vi "write_buffer_to_file.vi"(8 "error in (no error)":errorcluster, 10 "data_logger.lvclass":refnum<class "data_logger.lvclass">, 11 "tt20 in":refnum<class "tt20.lvclass">) -> (0 "error out":errorcluster, 1 "Stream_done":bool, 2 "data_logger.lvclass_out":refnum<class "data_logger.lvclass">, 3 "tt20 out":refnum<class "tt20.lvclass">)   [LabVIEW 2015, in "tt20.lvclass"]
uses:
  tt20.lvclass
  Data Logger Class/data_logger.lvclass
  tt20.lvclass/tt20.ctl
  C:/Users/MX-Microscope/Documents/LabVIEW Data/lvoop_campus_2018/Detector_Class/Swabian/time_tagger_vis/TTCSharp32.dll
  time_tagger_vis/TTCSharp32.dll
  lvoop_dll-master/picoquant_Tmodes.ctl
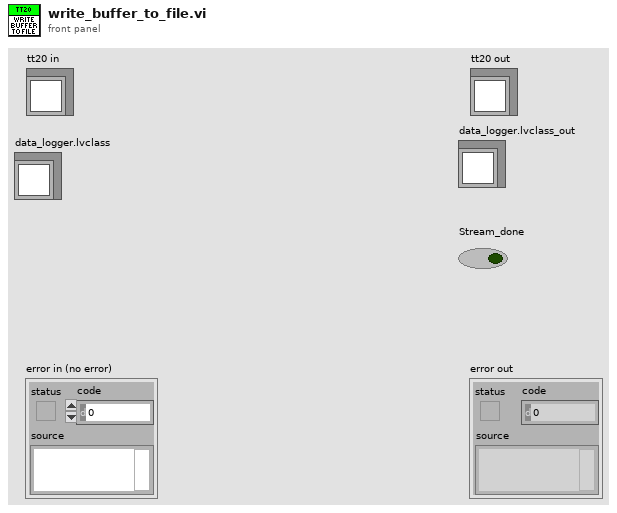
[diagram p1: front panel]
types:
  T1 = typedef "tt20_buffer_tdef.ctl" = cluster{"tagChannels":u32[], "tagTimestamps":i64[], "size":i32}
  T2 = typedef "picoquant_Tmodes.ctl" = u16
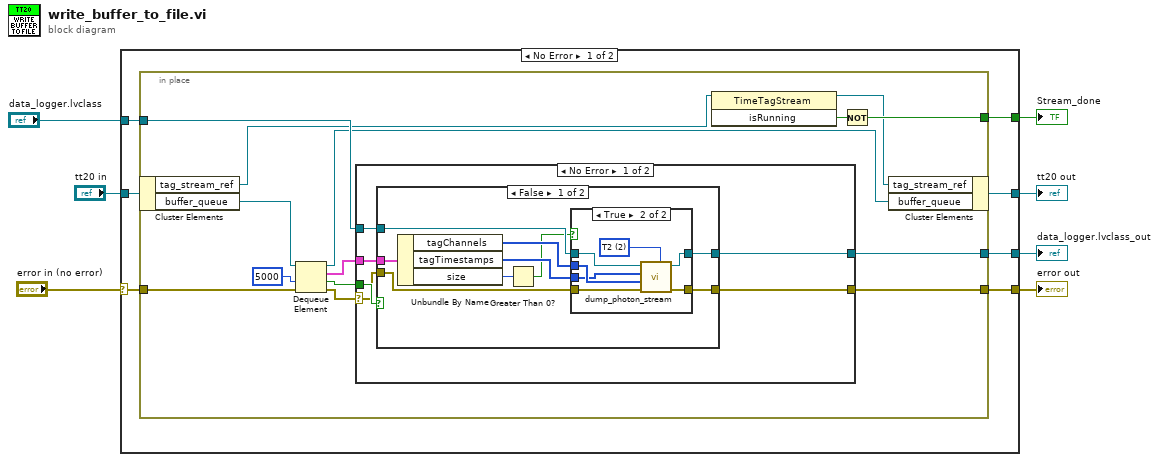
[diagram p0: block diagram]
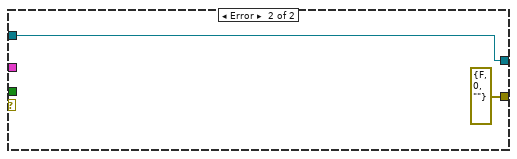
[diagram p4: hidden frame]
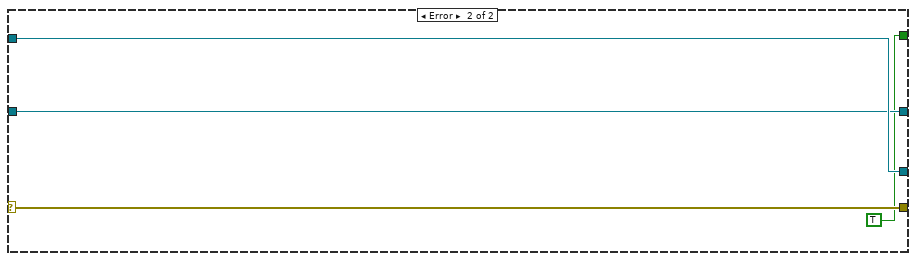
[diagram p5: hidden frame]
diagram:
  n1 = case shown="No Error" "error in (no error)" {
    selector: "error in (no error)" -> [w10 w60]
    tunnel: "tt20 in" -> [w14 w58]
    tunnel: [w13 w58] -> w5
    tunnel: "data_logger.lvclass" -> [w12 w59]
    tunnel: [w11 w59] -> w3
    tunnel: [w9 TRUE] -> w2
    tunnel: [w8 w60] -> w1
    frame No Error {
      n2 = in-place {
        in-place-border: w12 -> [w28]
        in-place-border: [w27] -> w11
        in-place-border: w10 -> [w25]
        in-place-border: [w18] -> w9
        in-place-border: [w17] -> w8
        n3 = in-place-cluster #1(w14) -> ("tag_stream_ref"=w20:refnum<k24>, "buffer_queue"=w26:refnum<queue>)
        n4 = Dequeue Element(queue=w26, timeout in ms (-1)=5000, error in (no error)=w25) -> (queue out=w21:refnum<queue>, element=w22:T1, timed out?=w23:bool, error out=w15:errorcluster)
        n5 = case shown="No Error" w15 {
          selector: w15 -> [w29 _]
          tunnel: w28 -> [w34 w56]
          tunnel: [w33 w56] -> w27
          tunnel: w23 -> [w32 _]
          tunnel: w22 -> [w31 _]
          tunnel: [w30 errorcluster {"status"=FALSE, "code"=0, "source"=""} ("error IO")] -> w17
          frame No Error {
            n6 = case shown="False" w32 {
              tunnel: w34 -> [w43 w53]
              tunnel: [w42 w53] -> w33
              tunnel: w29 -> [w41 w54]
              tunnel: w31 -> [w39 _]
              tunnel: [w40 w54] -> w30
              frame False {
                n7 = Unbundle By Name(w39) -> ("tagChannels"=w38:u32[], "tagTimestamps"=w37:i64[], "size"=w36:i32)
                n8 = Greater Than 0?(x=w36) -> (x > 0?=w35:bool)
                n9 = case shown="True" w35 {
                  tunnel: w43 -> [w45 w52]
                  tunnel: [w45 w51] -> w42
                  tunnel: w41 -> [w44 w49]
                  tunnel: [w44 w48] -> w40
                  tunnel: w38 -> [_ w47]
                  tunnel: w37 -> [_ w46]
                  frame False {
                  }
                  frame True {
                    w50 = T2 2 items=["T2"=2, "T3"=3] ("acq_mode")
                    n10 = call-dynamic "dump_photon_stream.vi"("Ring"=w50, "error in (no error)"=w49, "channels"=w47, "photon_records"=w46, "data_logger in"=w52) -> ("error out"=w48:errorcluster, "data_logger out"=w51:refnum<class "data_logger.lvclass">)  [unwired: 5 in]
                  }
                }
              }
              frame True {
              }
            }
          }
          frame Error {
          }
        }
        n11 = invoke class="TimeTagStream" method="isRunning"(reference=w20) -> (reference out=w16:refnum<k24>, "isRunning"=w19:bool)  [unwired: 2 in, 1 out]
        n12 = Not(x=w19) -> (.not. x?=w18:bool)
        n13 = in-place-cluster #1("tag_stream_ref"=w16, "buffer_queue"=w21) -> (w13:refnum<class "tt20.lvclass">)
      }
    }
    frame Error {
    }
  }
  "error out" <- w1
  "tt20 out" <- w5
  "data_logger.lvclass_out" <- w3
  "Stream_done" <- w2
